vi "Disabled.vi"(7 "Robot Mode":T2, 10 "Match Info":T1={"Autonomous Elapsed Seconds"=0.0, "TeleOp Elapsed Seconds"=0.0, "Disabled Elapsed Seconds"=0.0, "Visited Autonomous"=FALSE, "Visited TeleOp"=FALSE, "Visited Disabled"=FALSE, "Autonomous Settings"={"Autonomous Style"=enum."Independent", "VI Refnum"=refnum}}, 11 "Call Context":T3) -> ()   [LabVIEW 2014]
doc: "This VI is called each time a disabled packet is received from the DS. It is often used to prepare for the next robot mode, to calibrate sensors, etc."
uses:
  <vilib>/Rock Robotics/WPI/DriverStation/WPI_DriverStationDerivedRobotMode.ctl
  <vilib>/Rock Robotics/WPI/DriverStation/WPI_DriverStationRobotMode2.ctl
  <vilib>/Rock Robotics/WPI/DriverStation/WPI_DriverStationMatch Info.ctl
  Global Variables.vi
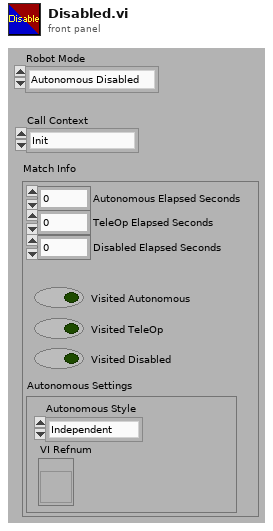
[diagram p1: front panel]
types:
  T1 = typedef "WPI_DriverStationMatch Info.ctl" = cluster{"Autonomous Elapsed Seconds":dbl, "TeleOp Elapsed Seconds":dbl, "Disabled Elapsed Seconds":dbl, "Visited Autonomous":bool, "Visited TeleOp":bool, "Visited Disabled":bool, "Autonomous Settings":cluster{"Autonomous Style":enum16{"Iterative", "Independent"}, "VI Refnum":refnum<vi>}}
  T2 = typedef "WPI_DriverStationRobotMode2.ctl" = enum16{"Autonomous Disabled", "Autonomous Enabled", "Teleop Disabled", "Teleop Enabled", "Disconnected", "Finish", "Test Disabled", "Test Enabled", "Emergency Stopped"}
  T3 = typedef "WPI_DriverStationDerivedRobotMode.ctl" = enum16{"Init", "Execute", "Stop"}
  T4 = typedef "WPI_CounterDevRef.ctl" = cluster{"DevStatus":errorcluster, "CntIndex":T5}
  T5 = typedef "FPGA_CounterCtrSystemIndex.ctl" = enum8{"Ctr 0", "Ctr 1", "Ctr 2", "Ctr 3", "Ctr 4", "Ctr 5", "Ctr 6", "Ctr 7", "Invalid"}
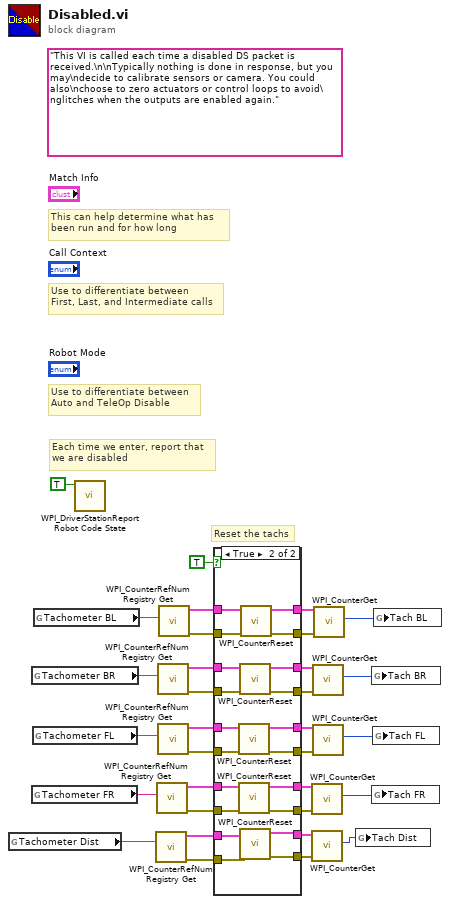
[diagram p0: block diagram]
diagram:
  (unwired) "This VI is called each time a disabled DS packet is received.\n\nTypically nothing is done in response, but you may\ndecide to calibrate sensors or camera. You could also\nchoose to zero actuators or control loops to avoid\nglitches when the outputs are enabled again."
  # "Reset the tachs"
  # "Each time we enter, report that\nwe are disabled"
  # "Use to differentiate between\nFirst, Last, and Intermediate calls"
  # "This can help determine what has\nbeen run and for how long"
  # "Use to differentiate between\nAuto and TeleOp Disable"
  n1 = global read "Global Variables.vi" "Tachometer Dist"() -> (w28:string)
  n2 = global read "Global Variables.vi" "Tachometer BR"() -> (w13:string)
  n3 = global read "Global Variables.vi" "Tachometer FR"() -> (w25:string)
  n4 = global read "Global Variables.vi" "Tachometer FL"() -> (w14:string)
  n5 = global read "Global Variables.vi" "Tachometer BL"() -> (w2:string)
  n6 = call <vilib>:"WPI_DriverStationReport Robot Code State.vi"("Disabled"=TRUE ("Autonomous")) -> ()  [unwired: 10 in, 1 out]
  n7 = call <vilib>:"WPI_CounterRefNum Registry Get.vi"("refnum name"=w28) -> ("error out"=w30:errorcluster, "CounterDevRef"=w26:T4)  [unwired: 9 in]
  n8 = call <vilib>:"WPI_CounterRefNum Registry Get.vi"("refnum name"=w25) -> ("error out"=w23:errorcluster, "CounterDevRef"=w24:T4)  [unwired: 9 in]
  n9 = call <vilib>:"WPI_CounterRefNum Registry Get.vi"("refnum name"=w13) -> ("error out"=w11:errorcluster, "CounterDevRef"=w12:T4)  [unwired: 9 in]
  n10 = call <vilib>:"WPI_CounterRefNum Registry Get.vi"("refnum name"=w14) -> ("error out"=w16:errorcluster, "CounterDevRef"=w15:T4)  [unwired: 9 in]
  n11 = call <vilib>:"WPI_CounterRefNum Registry Get.vi"("refnum name"=w2) -> ("error out"=w4:errorcluster, "CounterDevRef"=w3:T4)  [unwired: 9 in]
  n12 = case shown="True" TRUE {
    tunnel: w3 -> [w42 w62]
    tunnel: w4 -> [w41 w61]
    tunnel: [w42 w60] -> w5
    tunnel: [w41 w59] -> w6
    tunnel: w12 -> [w39 w49]
    tunnel: w11 -> [w40 w58]
    tunnel: [w39 w48] -> w10
    tunnel: [w40 w47] -> w9
    tunnel: w15 -> [w38 w50]
    tunnel: w16 -> [w37 w57]
    tunnel: [w38 w51] -> w17
    tunnel: [w37 w52] -> w18
    tunnel: w24 -> [w35 w55]
    tunnel: w23 -> [w36 w56]
    tunnel: [w35 w54] -> w22
    tunnel: [w36 w53] -> w21
    tunnel: w26 -> [w34 w46]
    tunnel: [w34 w45] -> w27
    tunnel: w30 -> [w33 w44]
    tunnel: [w33 w43] -> w31
    frame False {
    }
    frame True {
      n13 = call <vilib>:"WPI_CounterReset.vi"("error in (no error)"=w57, "CounterDevRef in"=w50) -> ("error out"=w52:errorcluster, "CounterDevRef out"=w51:T4)  [unwired: 8 in]
      n14 = call <vilib>:"WPI_CounterReset.vi"("error in (no error)"=w56, "CounterDevRef in"=w55) -> ("error out"=w53:errorcluster, "CounterDevRef out"=w54:T4)  [unwired: 8 in]
      n15 = call <vilib>:"WPI_CounterReset.vi"("error in (no error)"=w58, "CounterDevRef in"=w49) -> ("error out"=w47:errorcluster, "CounterDevRef out"=w48:T4)  [unwired: 8 in]
      n16 = call <vilib>:"WPI_CounterReset.vi"("error in (no error)"=w44, "CounterDevRef in"=w46) -> ("error out"=w43:errorcluster, "CounterDevRef out"=w45:T4)  [unwired: 8 in]
      n17 = call <vilib>:"WPI_CounterReset.vi"("error in (no error)"=w61, "CounterDevRef in"=w62) -> ("error out"=w59:errorcluster, "CounterDevRef out"=w60:T4)  [unwired: 8 in]
    }
  }
  n18 = call <vilib>:"WPI_CounterGet.vi"("error in (no error)"=w21, "CounterDevRef in"=w22) -> ("Value"=w20:i32)  [unwired: 4 in, 5 out]
  n19 = call <vilib>:"WPI_CounterGet.vi"("error in (no error)"=w31, "CounterDevRef in"=w27) -> ("Value"=w29:i32)  [unwired: 4 in, 5 out]
  n20 = call <vilib>:"WPI_CounterGet.vi"("error in (no error)"=w9, "CounterDevRef in"=w10) -> ("Value"=w8:i32)  [unwired: 4 in, 5 out]
  n21 = call <vilib>:"WPI_CounterGet.vi"("error in (no error)"=w18, "CounterDevRef in"=w17) -> ("Value"=w19:i32)  [unwired: 4 in, 5 out]
  n22 = call <vilib>:"WPI_CounterGet.vi"("error in (no error)"=w6, "CounterDevRef in"=w5) -> ("Value"=w7:i32)  [unwired: 4 in, 5 out]
  n23 = global write "Global Variables.vi" "Tach Dist"(w29) -> ()
  n24 = global write "Global Variables.vi" "Tach BR"(w8) -> ()
  n25 = global write "Global Variables.vi" "Tach FR"(w20) -> ()
  n26 = global write "Global Variables.vi" "Tach FL"(w19) -> ()
  n27 = global write "Global Variables.vi" "Tach BL"(w7) -> ()
